vi "SaveNewServerRef.vi"(2 "error":errorcluster, 3 "vi reference":refnum<vi>, 4 "Baxter in":T2) -> (0 "Active Topics":T1(array[cluster]), 1 "Baxter out":T2)   [LabVIEW 2010]
uses:
  <userlib>/ROSforLV_0.1/ROS/Code/SubVIs/_ROSControl.ctl
  <userlib>/ROSforLV_0.1/ROS/Code/SubVIs/_ROSDirection.ctl
  <userlib>/ROSforLV_0.1/ROS/Code/_ROSDefinition.vi
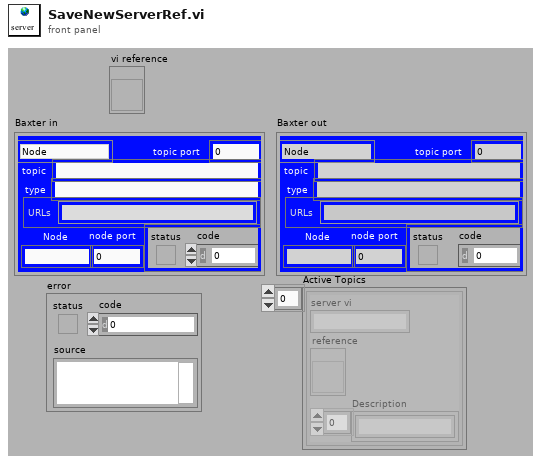
[diagram p1: front panel]
types:
  T1 = cluster{"server vi":string, "reference":refnum<vi>, "Description":string[]}[]
  T2 = typedef "_ROSControl.ctl" = cluster{"topic port":u16, "Node":string, "topic":string, "type":string, "node port":u32, "error ":errorcluster, "Direction":T3, "APIs":string[]}
  T3 = typedef "_ROSDirection.ctl" = enum16{"Node", "Publisher", "Subscriber", "Service Client"}
  T4 = cluster{"vi name":string, "vi reference":refnum<vi>, string[]}
  T5 = cluster{"vi name":string, "vi reference":refnum<vi>, "Description":string[]}[]
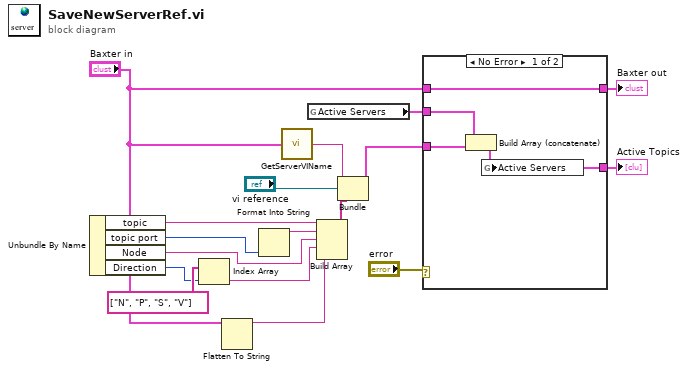
[diagram p0: block diagram]
diagram:
  n1 = Unbundle By Name("Baxter in") -> ("topic"=w6:string, "topic port"=w12:u16, "Node"=w7:string, "Direction"=w9:T3)
  n2 = Index Array(array=string[] ["N", "P", "S", "V"], index=w9) -> (element=w8:string)
  n3 = Flatten To String(anything="Baxter in") -> (data string=w1:string)  [unwired: 3 in, 2 out]
  n4 = Format Into String(w12) -> (resulting string=w11:string)  [unwired: 3 in, 1 out]
  n5 = call <userlib>:"GetServerVIName.vi"("Baxter"="Baxter in") -> ("vi name"=w15:string)
  n6 = global read "_ROSDefinition.vi" "Active Servers"() -> (w3:T1)
  n7 = Build Array(w6, w11, w7, w8, w1) -> (w5:string[])
  n8 = Bundle("vi name"=w15, "vi reference"="vi reference", w5) -> (w13:T4)  [unwired: 1 in]
  n9 = case shown="No Error" "error" {
    tunnel: [w20 w23] -> w16
    tunnel: "Baxter in" -> [w20 w23]
    tunnel: w13 -> [w21 _]
    tunnel: [w19 w22] -> w4
    tunnel: w3 -> [w18 w22]
    frame No Error {
      n10 = Build Array (concatenate)(w18, w21) -> (w19:T5)
      n11 = global write "_ROSDefinition.vi" "Active Servers"(w19) -> ()
    }
    frame Error {
    }
  }
  "Baxter out" <- w16
  "Active Topics" <- w4
